vi "INIT.vi"(8 "error in (no error)":errorcluster, 11 "UI Actor in":refnum<class "UI Actor.lvclass">) -> (0 "error out":errorcluster, 3 "UI Actor out":refnum<class "UI Actor.lvclass">)   [LabVIEW 2019, in "UI Actor.lvlib" / "UI Actor.lvclass"]
uses:
  UI Actor.lvclass
  C:/Program Files (x86)/National Instruments/LabVIEW 2019/vi.lib/ActorFramework/Actor/Actor.lvclass
  UI Actor.lvclass/UI Actor.ctl
  MXN ACTOR/MXN ACTOR.lvclass
  MXN ACTOR/MXN ACTOR.lvclass/MXN ACTOR.ctl
  USD ACTOR/USD ACTOR.lvclass
  USD ACTOR/USD ACTOR.lvclass/USD ACTOR.ctl
  Read Coins.vi
  Read Sub panel coin.vi
  <vilib>/ActorFramework/Actor/Actor.lvclass
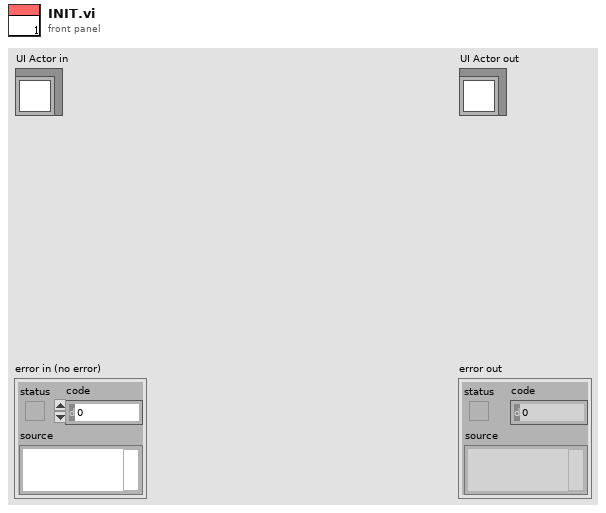
[diagram p1: front panel]
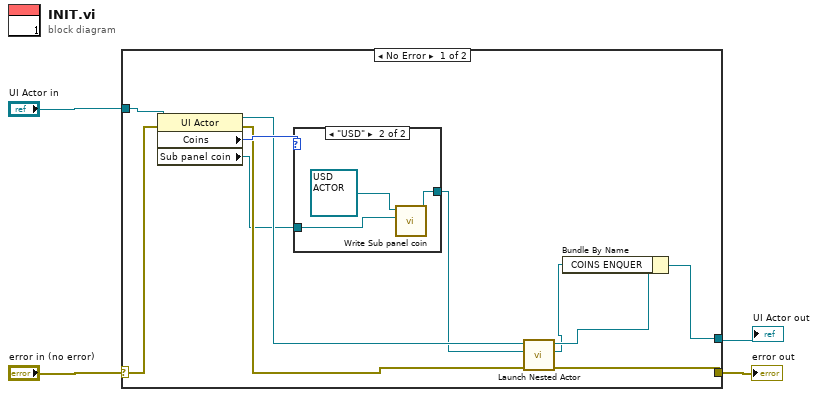
[diagram p0: block diagram]
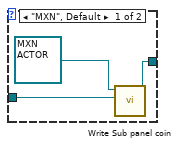
[diagram p2: hidden frame]
diagram:
  n1 = case shown="No Error" "error in (no error)" {
    selector: "error in (no error)" -> [w14 w23]
    tunnel: [w11 w23] -> w3
    tunnel: [w8 w22] -> w1
    tunnel: "UI Actor in" -> [w15 w22]
    frame No Error {
      n2 = property class="UI Actor"(reference=w15, error in=w14) -> (reference out=w10:refnum<class "UI Actor.lvclass">, error out=w12:errorcluster, "Coins"=w13:enum16{"MXN", "USD", ""}, "Sub panel coin"=w5:refnum<vi>)
      n3 = case shown="\"USD\"" w13 {
        tunnel: [w17 w19] -> w9
        tunnel: w5 -> [w16 w20]
        frame "MXN", Default {
          n4 = call "Write Sub panel coin.vi"("Sub panel coin"=w16, "MXN ACTOR in"=refnum<class "MXN ACTOR.lvclass"> refnum ("MXN ACTOR.lvlib:MXN ACTOR.lvclass")) -> ("MXN ACTOR out"=w17:refnum<class "MXN ACTOR.lvclass">)  [unwired: 8 in, 1 out]
        }
        frame "USD" {
          n5 = call "Write Sub panel coin.vi"("Sub panel coin"=w20, "USD ACTOR in"=refnum<class "USD ACTOR.lvclass"> refnum ("USD ACTOR.lvlib:USD ACTOR.lvclass")) -> ("USD ACTOR out"=w19:refnum<class "USD ACTOR.lvclass">)  [unwired: 8 in, 1 out]
        }
      }
      n6 = call <vilib>:"Launch Nested Actor.vi"("error in (no error)"=w12, "Nested Actor"=w9, "Caller Actor in"=w10) -> ("error out"=w11:errorcluster, "Nested Actor's Enqueuer"=w6:refnum<class "Message Enqueuer.lvclass">, "Caller Actor out"=w7:refnum<class "UI Actor.lvclass">)  [unwired: 6 in]
      n7 = Bundle By Name(cluster=w7, "COINS ENQUER"=w6) -> (w8:refnum<class "UI Actor.lvclass">)
    }
    frame Error {
    }
  }
  "error out" <- w3
  "UI Actor out" <- w1
